vi "R1C_Att_To_Bit.vi"(1 "Att":T1 items=["0.0", "0.5", "1.0", "1.5", "2.0", "2.5", "3.0", "3.5", "4.0", "4.5", "5.0", "5.5", "6.0", "6.5", "7.0", "7.5", "8.0", "8.5", "9.0", "9.5", "10.0", "10.5", "11.0", "11.5", "12.0", "12.5", "13.0", "13.5", "14.0", "14.5", "15.0", "15.5", "16.0", "16.5", "17.0", "17.5", "18.0", "18.5", "19.0", "19.5", "20.0", "20.5", "21.0", "21.5", "22.0", "22.5", "23.0", "23.5", "24.0", "24.5", "25.0", "25.5", "26.0", "26.5", "27.0", "27.5", "28.0", "28.5", "29.0", "29.5", "30.0", "30.5", "31.0", "31.5"]) -> (0 "Bit":u32 caption="bit" format="%b")   [LabVIEW 2018]
uses:
  Types/Att(0-0.5-31.5).ctl
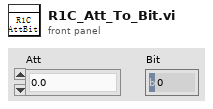
[diagram p1: front panel]
types:
  T1 = typedef "Att(0-0.5-31.5).ctl" = dbl
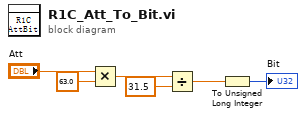
[diagram p0: block diagram]
diagram:
  n1 = Multiply(x="Att", y=63.0) -> (x*y=w4:T1)
  n2 = Divide(x=w4, y=31.5) -> (x/y=w2:T1)
  n3 = To Unsigned Long Integer(number=w2) -> (unsigned 32bit integer=→"Bit":u32)
